vi "_PC_Pub_RecipeFormatString_SearchVariable.vi"(10 "VarName":string, 11 "String_in":string="VarName") -> (0 "No found":bool, 1 "Var":string, 2 "Var":dbl, 3 "String_out":string)   [LabVIEW 2018]
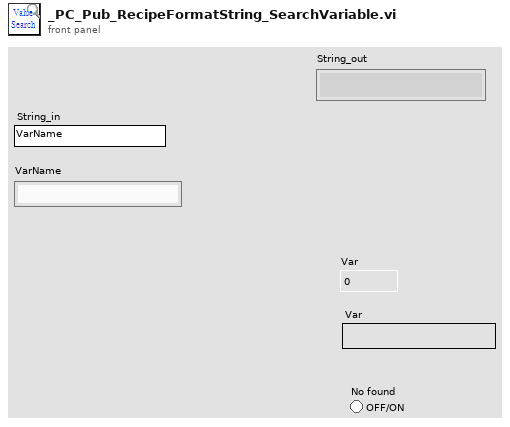
[diagram p1: front panel]
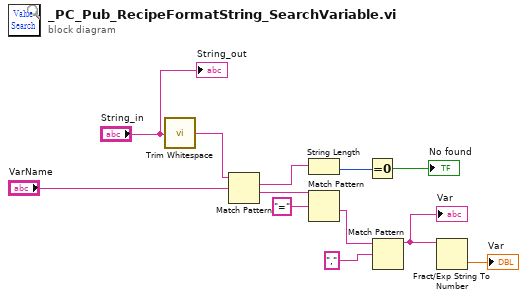
[diagram p0: block diagram]
diagram:
  n1 = call <vilib>:"Trim Whitespace.vi"("string"="String_in") -> ("trimmed string"=w8:string)  [unwired: 1 in]
  n2 = Match Pattern(string=w8, regular expression="VarName") -> (match substring=w7:string, after substring=w12:string)  [unwired: 1 in, 2 out]
  n3 = String Length(string=w7) -> (length=w6:i32)
  n4 = Match Pattern(string=w12, regular expression="=") -> (after substring=w10:string)  [unwired: 1 in, 3 out]
  n5 = Equal To 0?(x=w6) -> (x = 0?=→"No found":bool)
  n6 = Match Pattern(string=w10, regular expression=",") -> (before substring=w4:string)  [unwired: 1 in, 3 out]
  "Var" <- w4
  n7 = Fract/Exp String To Number(string=w4) -> (number=→"Var":dbl)  [unwired: 3 in, 1 out]
  "String_out" <- "String_in"
